vi "总磷总氮质控参数设置.vi"(11 "质控参数设置":T1) -> (2 "质控参数设置 2":T1, 3 "check？":bool)   [LabVIEW 2016, in "斯坦道通用流路CODmn.lvlib"]
uses:
  <vilib>/Utility/miscctls.llb/LVPointTypeDef.ctl
panel:
  in  "质控参数":i32(listbox)
  in  "取消":bool
  in  "确定":bool
  # "质控参数设置"
  # "质控参数设置"
  # "总氮"
  # "COD"
  # "氨氮"
  # "监测参数"
  # "总磷"
  # "跨度值"
  # "零点核查标准液浓度"
  # "跨度核查标准液浓度"
  # "标样核查标准液浓度"
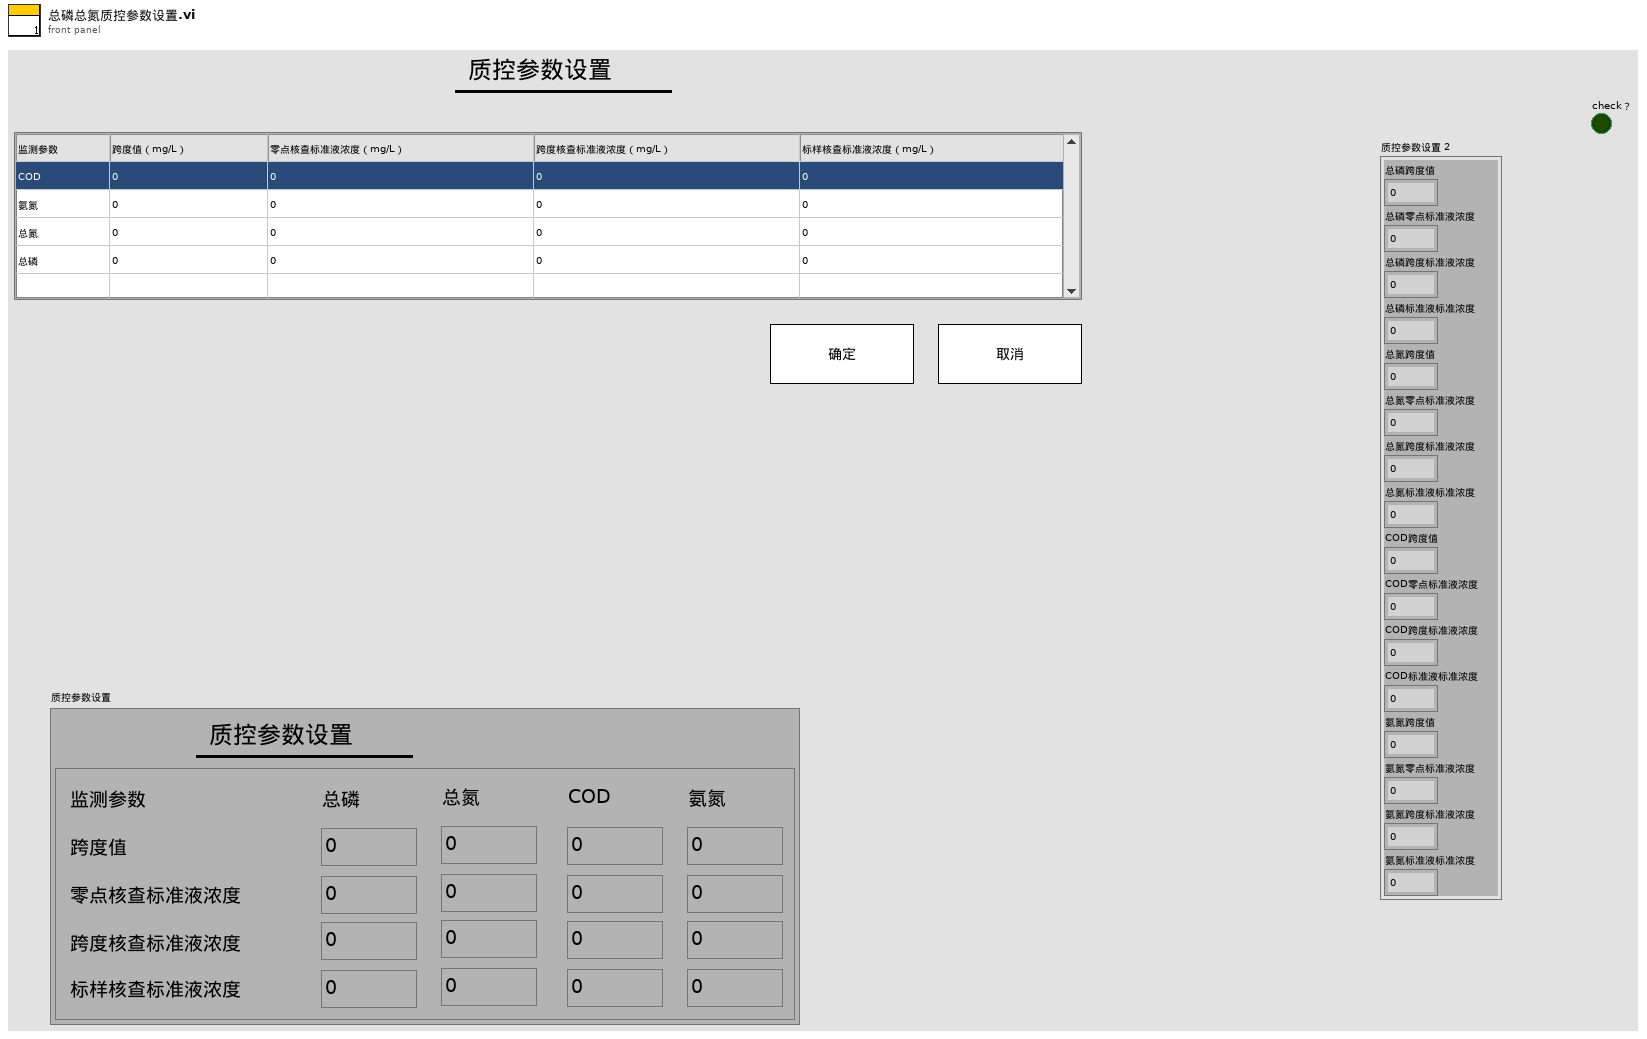
[diagram p1: front panel]
types:
  T1 = cluster{"总磷跨度值":dbl, "总磷零点标准液浓度":dbl, "总磷跨度标准液浓度":dbl, "总磷标准液标准浓度":dbl, "总氮跨度值":dbl, "总氮零点标准液浓度":dbl, "总氮跨度标准液浓度":dbl, "总氮标准液标准浓度":dbl, "COD跨度值":dbl, "COD零点标准液浓度":dbl, "COD跨度标准液浓度":dbl, "COD标准液标准浓度":dbl, "氨氮跨度值":dbl, "氨氮零点标准液浓度":dbl, "氨氮跨度标准液浓度":dbl, "氨氮标准液标准浓度":dbl}
  T2 = typedef "LVPointTypeDef.ctl" = cluster{"Horizontal":i16, "Vertical":i16}
  T3 = typedef "LVPoint32TypeDef.ctl" = cluster{"Horizontal":i32, "Vertical":i32}
  T4 = typedef "LVRowAndColumnTypeDef.ctl" = cluster{"Row":i32, "Column":i32}
  T5 = cluster{"质控参数设置[0]":dbl, "质控参数设置[1]":dbl, "质控参数设置[2]":dbl, "质控参数设置[3]":dbl, "质控参数设置[4]":dbl, "质控参数设置[5]":dbl, "质控参数设置[6]":dbl, "质控参数设置[7]":dbl, "质控参数设置[8]":dbl, "质控参数设置[9]":dbl, "质控参数设置[10]":dbl, "质控参数设置[11]":dbl, "质控参数设置[12]":dbl, "质控参数设置[13]":dbl, "质控参数设置[14]":dbl, "质控参数设置[15]":dbl}
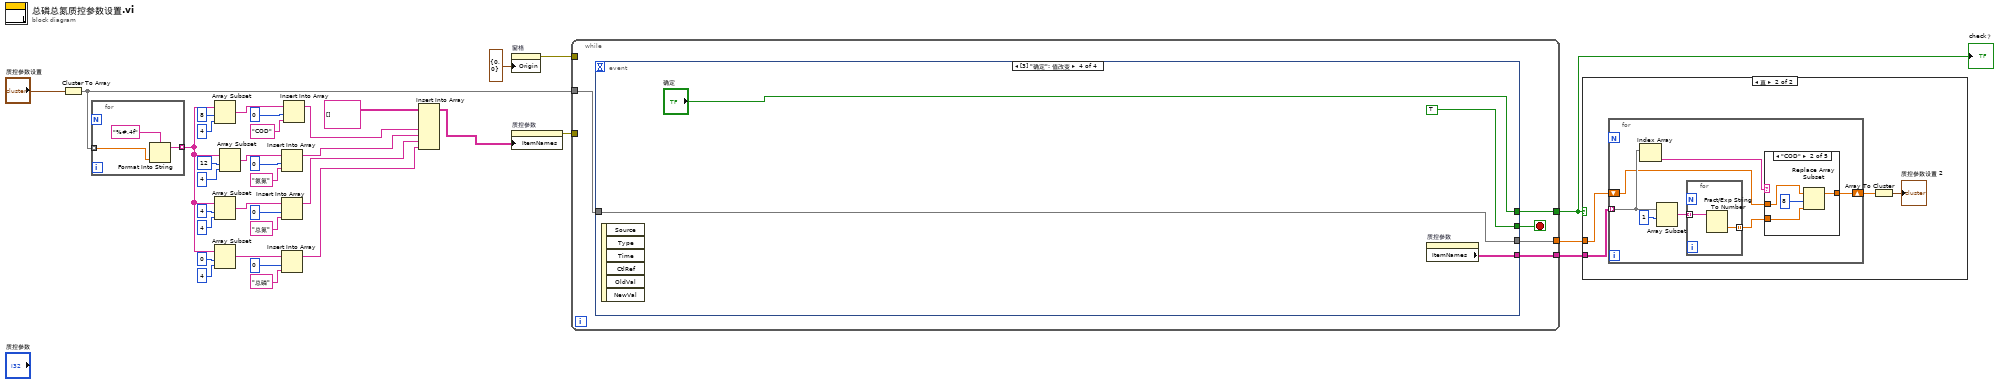
[diagram p0: block diagram]
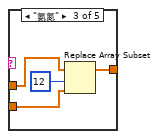
[diagram p4: hidden frame]
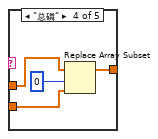
[diagram p5: hidden frame]
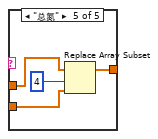
[diagram p6: hidden frame]
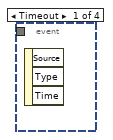
[diagram p7: hidden frame]
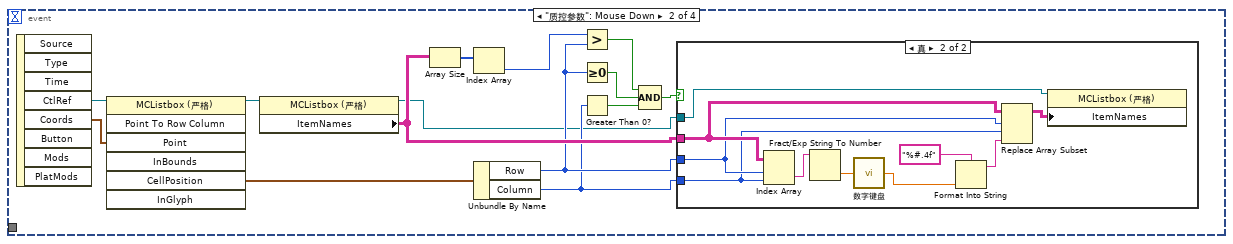
[diagram p8: hidden frame]
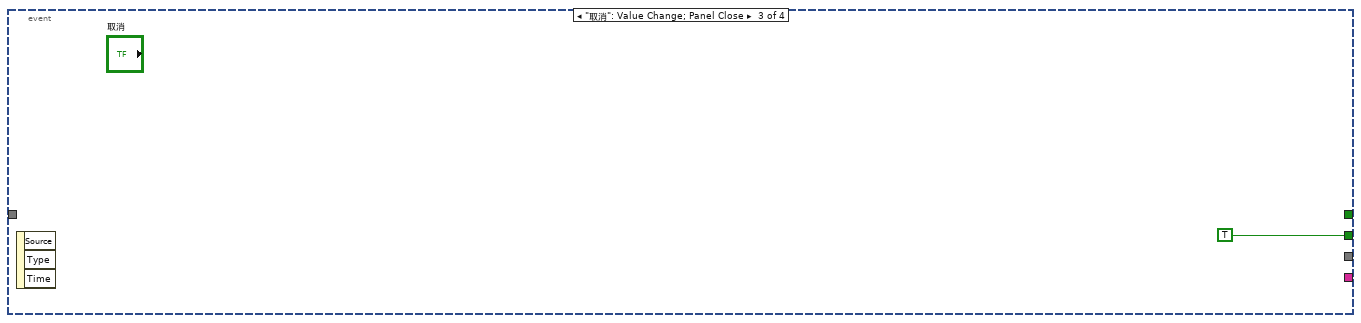
[diagram p10: hidden frame]
diagram:
  n1 = Cluster To Array(cluster="质控参数设置") -> (array=w4:dbl[])
  n2 = for {
    tunnel: w4 -> [w37] mode=indexing
    tunnel: [w36] -> w12 mode=indexing
    n3 = Format Into String(format string="%#.4f" ("格式字符串"), w37) -> (resulting string=w36:string)  [unwired: 2 in, 1 out]
  }
  n4 = Array Subset(array=w12, index=8 ("索引"), length=4 ("长度")) -> (w20:string[])
  n5 = Array Subset(array=w12, index=4 ("索引"), length=4 ("长度")) -> (w25:string[])
  n6 = Array Subset(array=w12, index=0 ("索引"), length=4 ("长度")) -> (w30:string[])
  n7 = Array Subset(array=w12, index=12 ("索引"), length=4 ("长度")) -> (w15:string[])
  n8 = Insert Into Array(array=w15, index=0 ("索引"), new element="氨氮" ("新元素/子数组")) -> (w9:string[])
  n9 = Insert Into Array(array=w25, index=0 ("索引"), new element="总氮" ("新元素/子数组")) -> (w8:string[])
  n10 = Insert Into Array(array=w30, index=0 ("索引"), new element="总磷" ("新元素/子数组")) -> (w7:string[])
  n11 = Insert Into Array(array=w20, index=0 ("索引"), new element="COD" ("新元素/子数组")) -> (w10:string[])
  n12 = Insert Into Array(array=string[][] [], new element #1=w10, new element #2=w9, new element #3=w8, new element #4=w7) -> (w5:string[][])  [unwired: 2 in]
  n13 = property on="窗格" class="Pane"("Origin"=T2 {"Horizontal"=0, "Vertical"=0} ("原点")) -> (error out=w34:errorcluster)  [unwired: 2 in, 1 out]
  n14 = property on="质控参数" class="MCListbox (严格)"("ItemNames"=w5) -> (error out=w6:errorcluster)  [unwired: 2 in, 1 out]
  n15 = while {
    tunnel: w34 -> [_]
    tunnel: [w42] -> w1
    tunnel: w6 -> [_]
    tunnel: w4 -> [w41]
    tunnel: [w40] -> w3
    tunnel: [w39] -> w2
    stop <- w43 stop-if-true
    n16 = event shown="[3] \"确定\": 值改变" {
      selector: _ -> [_ _ _ _]
      dyn-events: _ -> [_ _ _ _]
      timeout: _ -> [_ _ _ _]
      tunnel: [_ _ TRUE TRUE] -> w43
      tunnel: [_ _ _ "确定"] -> w42
      tunnel: w41 -> [_ _ _ w70]
      tunnel: [_ _ _ w70] -> w40
      tunnel: [_ _ _ w69] -> w39
      event Timeout {
        n17 = event-data() -> ()  [unwired: 1 in, 3 out]
      }
      event "质控参数": Mouse Down {
        n18 = event-data() -> ("CtlRef"=w57:refnum<vi>, "Coords"=w56:T3)  [unwired: 1 in, 6 out]
        n19 = invoke class="MCListbox (严格)" method="Point To Row Column"(reference=w57, "Point"=w56) -> (reference out=w55:refnum<vi>, "CellPosition"=w54:T4)  [unwired: 5 in, 5 out]
        n20 = property class="MCListbox (严格)"(reference=w55) -> (reference out=w44:refnum<vi>, "ItemNames"=w47:string[][])  [unwired: 1 in, 1 out]
        n21 = Array Size(array=w47) -> (size(s)=w51:i32[])
        n22 = Index Array(array=w51) -> (element=w50:i32)  [unwired: 1 in]
        n23 = Unbundle By Name(w54) -> ("Row"=w46:i32, "Column"=w45:i32)
        n24 = Greater?(x=w50, y=w46) -> (0:w49:bool)
        n25 = Greater Or Equal To 0?(x=w46) -> (x >= 0?=w48:bool)
        n26 = Greater Than 0?(x=w45) -> (x > 0?=w53:bool)
        n27 = Compound Arithmetic op=AND ("复合运算")(w49, w48, w53) -> (w52:bool)
        n28 = case shown="真" w52 {
          tunnel: w47 -> [_ w63]
          tunnel: w46 -> [_ w62]
          tunnel: w45 -> [_ w61]
          tunnel: w44 -> [_ w58]
          frame False {
          }
          frame True {
            n29 = Index Array(array=w63, index (row)=w62, index (col)=w61) -> (element=w67:string)
            n30 = Fract/Exp String To Number(string=w67) -> (number=w66:dbl)  [unwired: 3 in, 1 out]
            n31 = call "数字键盘.vi"("OldNumber"=w66) -> ("NewNumber"=w65:dbl)
            n32 = Format Into String(format string="%#.4f" ("格式字符串"), w65) -> (resulting string=w60:string)  [unwired: 2 in, 1 out]
            n33 = Replace Array Subset(array=w63, new element=w60, index (row)=w62, index (col)=w61) -> (w59:string[][])
            n34 = property class="MCListbox (严格)"(reference=w58, "ItemNames"=w59) -> ()  [unwired: 1 in, 2 out]
          }
        }
      }
      event "取消": Value Change; Panel Close {
        n35 = event-data() -> ()  [unwired: 1 in, 3 out]
      }
      event "确定": Value Change {
        n36 = event-data() -> ()  [unwired: 1 in, 6 out]
        n37 = property on="质控参数" class="MCListbox (严格)"() -> ("ItemNames"=w69:string[][])  [unwired: 2 in, 2 out]
      }
    }
  }
  "check？" <- w1
  n38 = case shown="真" w1 {
    tunnel: w3 -> [_ w76]
    tunnel: w2 -> [_ w75]
    frame False {
    }
    frame True {
      n39 = for {
        tunnel: w75 -> [w82] mode=indexing
        shift-right: [w77] -> w74
        shift-left: w76 -> [w78]
        n40 = Index Array(array=w82) -> (element=w83:string)  [unwired: 1 in]
        n41 = Array Subset(array=w82, index=1 ("索引")) -> (w80:string[])  [unwired: 1 in]
        n42 = for {
          tunnel: w80 -> [w85] mode=indexing
          tunnel: [w84] -> w79 mode=indexing
          n43 = Fract/Exp String To Number(string=w85) -> (number=w84:dbl)  [unwired: 3 in, 1 out]
        }
        n44 = case shown="\"COD\"" w83 {
          tunnel: w79 -> [_ w89 w93 w97 w101]
          tunnel: w78 -> [w86 w90 w94 w98 w102]
          tunnel: [w86 w88 w92 w96 w100] -> w77
          frame Default {
          }
          frame "COD" {
            n45 = Replace Array Subset(array=w90, new element=w89, index=8 ("索引")) -> (w88:dbl[])
          }
          frame "氨氮" {
            n46 = Replace Array Subset(array=w94, new element=w93, index=12 ("索引")) -> (w92:dbl[])
          }
          frame "总磷" {
            n47 = Replace Array Subset(array=w98, new element=w97, index=0 ("索引")) -> (w96:dbl[])
          }
          frame "总氮" {
            n48 = Replace Array Subset(array=w102, new element=w101, index=4 ("索引")) -> (w100:dbl[])
          }
        }
      }
      n49 = Array To Cluster(array=w74) -> (cluster=→"质控参数设置 2":T5)
    }
  }
